vi "Application User Name.vi"(8 "Error In":errorcluster) -> (0 "Error Out":errorcluster, 3 "User Name":string)   [LabVIEW 2017, in "Toolkit VIs.lvlib"]
uses:
  Toolkit VIs.lvlib
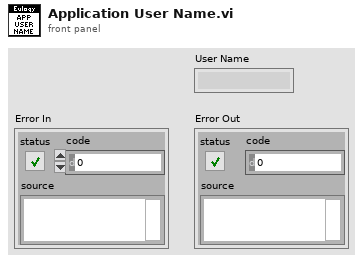
[diagram p1: front panel]
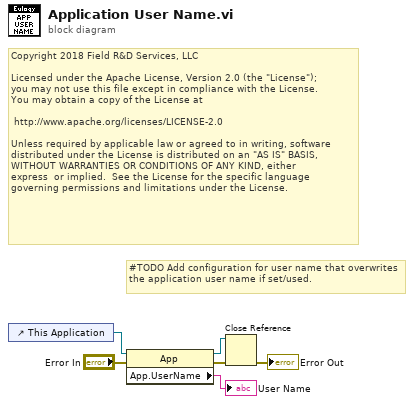
[diagram p0: block diagram]
diagram:
  # "Copyright 2018 Field R&D Services, LLC\n\nLicensed under the Apache License, Version 2.0 (the \"License\");\nyou may not use this file except in compliance with the License.\nYou may obtain a copy of the License at\n\n\thttp://www.apache.org/licenses/LICENSE-2.0\n\nUnless required by applicable law or agreed to in writing, software\ndistributed under the License is distributed on an \"AS IS\" BASIS,\nWITHOUT WARRANTIES OR CONDITIONS OF ANY KIND, either \nexpress  or implied.  See the License for the specific language \ngoverning permissions and limitations under the License."
  # "#TODO Add configuration for user name that overwrites the application user name if set/used."
  n1 = control-ref of="This Application"() -> (w1:refnum<vi>)
  n2 = property class="App"(reference=w1, error in="Error In") -> (reference out=w6:refnum<vi>, error out=w3:errorcluster, "App.UserName"=→"User Name":string)
  n3 = Close Reference(reference=w6, error in (no error)=w3) -> (error out=→"Error Out":errorcluster)
